vi "PropertyChangedEventCallbackForCameraState.vi"(4 "Cluster":T2, 5 "Event Data":cluster{"sender":refnum<k24>, "e":refnum<k24>}, 6 "Control Ref":refnum<k24>, 7 "Event Common Data":T3) -> ()   [LabVIEW 2019]
uses:
  D:/SDK/PMQI-LabViewSamples/Examples/Dependencies/PVCamNET.dll
  controls/UI Data.ctl
  support/Message Queue/Message Cluster.ctl
  support/Message Queue/Enqueue Message (Single).vi
  support/Message Queue/Message Queue.lvlib
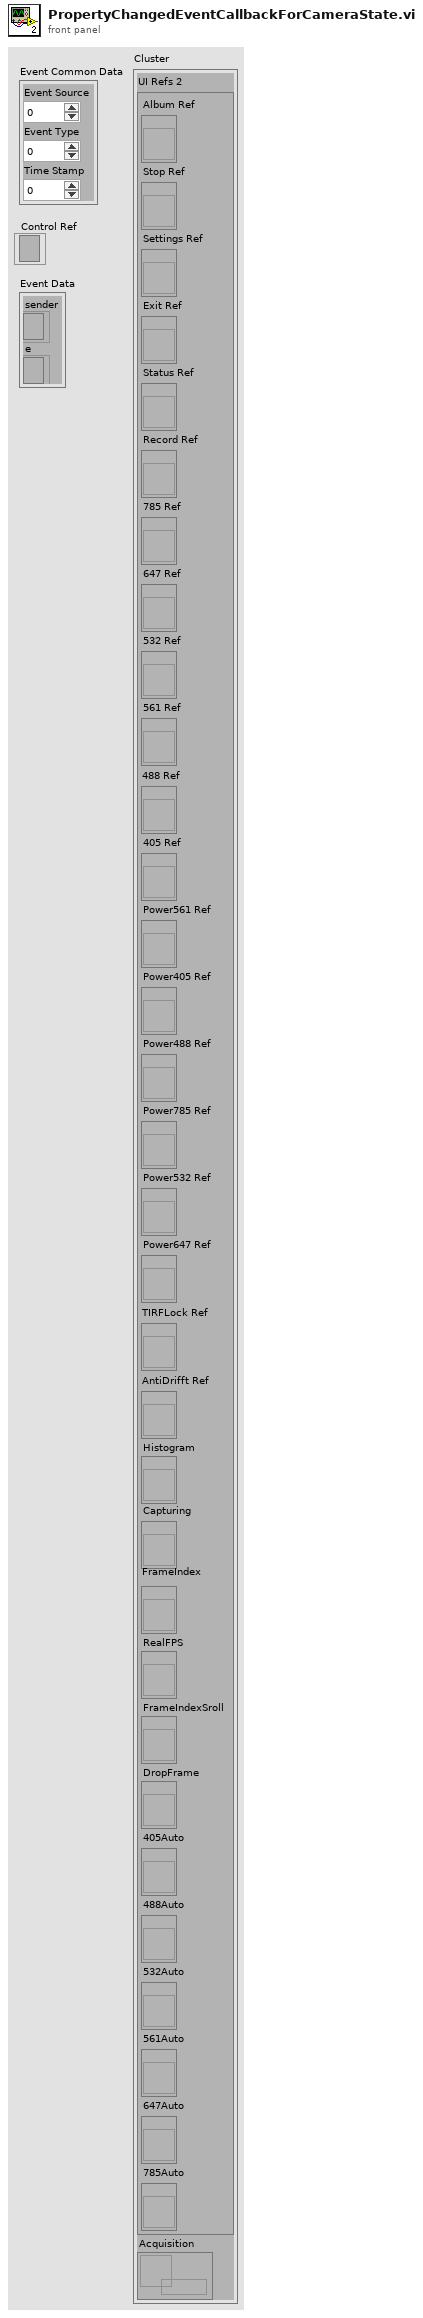
[diagram p1: front panel]
types:
  T1 = typedef "UI Data.ctl" = cluster{"Album Ref":refnum<vi>, "Stop Ref":refnum<vi>, "Settings Ref":refnum<vi>, "Exit Ref":refnum<vi>, "Status Ref":refnum<vi>, "Record Ref":refnum<vi>, "785 Ref":refnum<vi>, "647 Ref":refnum<vi>, "532 Ref":refnum<vi>, "561 Ref":refnum<vi>, "488 Ref":refnum<vi>, "405 Ref":refnum<vi>, "Power561 Ref":refnum<vi>, "Power405 Ref":refnum<vi>, "Power488 Ref":refnum<vi>, "Power785 Ref":refnum<vi>, "Power532 Ref":refnum<vi>, "Power647 Ref":refnum<vi>, "TIRFLock Ref":refnum<vi>, "AntiDrifft Ref":refnum<vi>, "Histogram":refnum<vi>, "Capturing":refnum<vi>, "FrameIndex":refnum<vi>, "RealFPS":refnum<vi>, "FrameIndexSroll":refnum<vi>, "DropFrame":refnum<vi>, "405Auto":refnum<vi>, "488Auto":refnum<vi>, "532Auto":refnum<vi>, "561Auto":refnum<vi>, "647Auto":refnum<vi>, "785Auto":refnum<vi>}
  T2 = cluster{"UI Refs 2":T1, "Acquisition":refnum<queue>}
  T3 = cluster{"Event Source":i32, "Event Type":u32, "Time Stamp":u32}
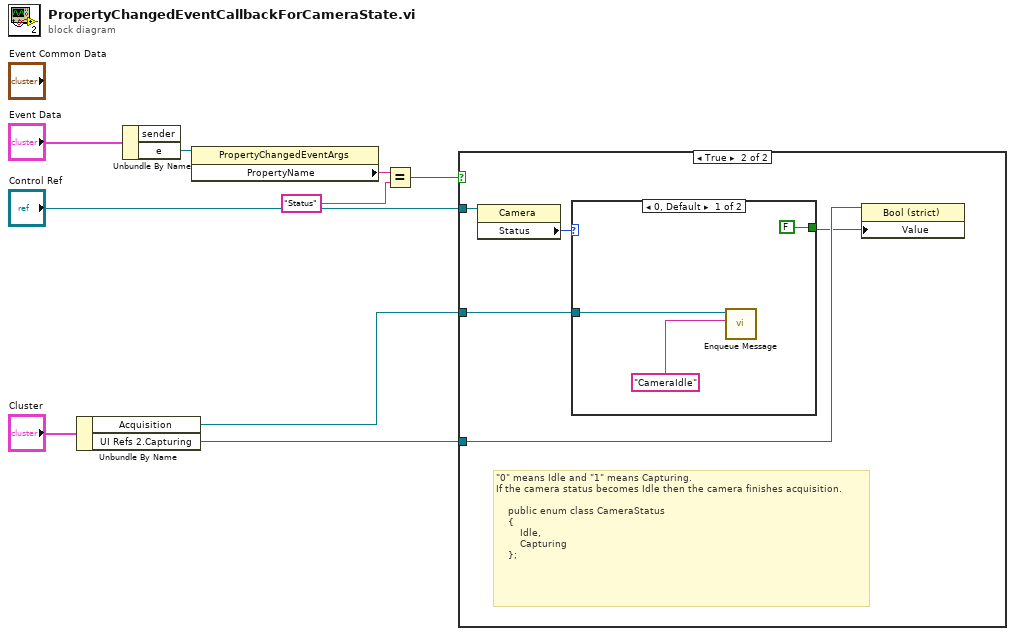
[diagram p0: block diagram]
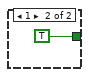
[diagram p3: hidden frame]
diagram:
  n1 = Unbundle By Name("Cluster") -> ("Acquisition"=w1:refnum<queue>, "UI Refs 2.Capturing"=w2:refnum<vi>)
  n2 = Unbundle By Name("Event Data") -> ("e"=w9:refnum<k24>)  [unwired: 1 out]
  n3 = property class="PropertyChangedEventArgs"(reference=w9) -> ("PropertyName"=w8:string)  [unwired: 1 in, 2 out]
  n4 = Equal?(x=w8, y="Status") -> (x = y?=w6:bool)
  n5 = case shown="True" w6 {
    tunnel: w2 -> [_ w12]
    tunnel: "Control Ref" -> [_ w14]
    tunnel: w1 -> [_ w10]
    frame False {
    }
    frame True {
      # "\"0\" means Idle and \"1\" means Capturing.\nIf the camera status becomes Idle then the camera finishes acquisition.\n\n    public enum class CameraStatus\n    {\n        Idle,\n        Capturing\n    };"
      n6 = property class="Camera"(reference=w14) -> ("Status"=w13:i32)  [unwired: 1 in, 2 out]
      n7 = case shown="0, Default" w13 {
        tunnel: [FALSE TRUE] -> w11
        tunnel: w10 -> [w15 _]
        frame 0, Default {
          n8 = call-poly "Enqueue Message.vi"("Message"="CameraIdle", "Message Queue"=w15) -> ()  [unwired: 8 in, 2 out]
        }
        frame 1 {
        }
      }
      n9 = property class="Bool (strict)"(reference=w12, "Value"=w11) -> ()  [unwired: 1 in, 2 out]
    }
  }
